vi "SubVI_IntakePID_teleop.vi"(10 "output range":cluster{"output high":dbl, "output low":dbl}={"output high"=100.0, "output low"=-100.0} {"output low" format="%.2f"; "output high" format="%.2f"}, 11 "PID gains":T1={"proportional gain (Kc)"=1.0, "integral time (Ti, min)"=0.01, "derivative time (Td, min)"=0.0} {"derivative time (Td, min)" format="%.3f"; "integral time (Ti, min)" format="%.3f"; "proportional gain (Kc)" format="%.3f"}) -> ()   [LabVIEW 2017]
uses:
  <vilib>/Rock Robotics/Network Tables/NT Read Number.vi
  <vilib>/addons/control/pid/pid.llb/PID (DBL).vi
  <vilib>/addons/control/pid/NI_PID_pid.lvlib
panel:
  out "x-y":dbl
  out "PIDF output":dbl format="%.2f"
  out "Encoder value":dbl
  out "encoder value/PID output":cluster{"output":dbl, "Distance":dbl, dbl}(graph)
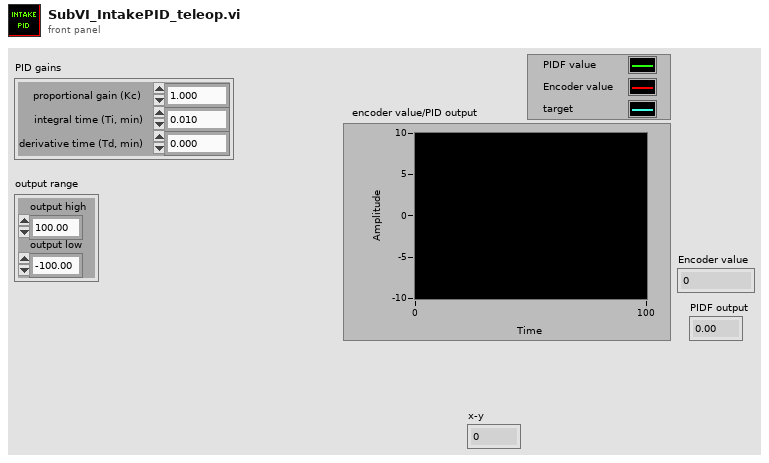
[diagram p1: front panel]
types:
  T1 = cluster{"proportional gain (Kc)":dbl, "integral time (Ti, min)":dbl, "derivative time (Td, min)":dbl}
  T2 = typedef "WPI_EncoderDevRef.ctl" = cluster{"DevStatus":errorcluster, "EncoderIndex":T3, "CounterIndex":T4, "DistancePerCount":dbl, "Decoding Type":T5}
  T3 = typedef "FPGA_EncoderIdx.ctl" = enum8{"Enc 0", "Enc 1", "Enc 2", "Enc 3", "Enc 4", "Enc 5", "Enc 6", "Enc 7", "Invalid"}
  T4 = typedef "FPGA_CounterCtrSystemIndex.ctl" = enum8{"Ctr 0", "Ctr 1", "Ctr 2", "Ctr 3", "Ctr 4", "Ctr 5", "Ctr 6", "Ctr 7", "Invalid"}
  T5 = typedef "WPI_EncoderType.ctl" = enum16{"1x", "2x", "4x"}
  T6 = typedef "WPI_MotorControlDeviceRef.ctl" = cluster{"DeviceStatus":errorcluster, "Type":T7, "PWM":cluster{"PWM Channel":T8, "DeadBand":T9}, "CAN":cluster{"Device Number":u8, "SetOutput VI Ref":variant, "GetOutput VI Ref":variant, "Enable VI Ref":variant, "Disable VI Ref":variant, "Data":variant}, "Invert":bool, "DIO PWM":cluster{"PWM \"Enable\" Channel":T8, "DIOChannel":T10, "PWM Rate":dbl}}
  T7 = typedef "WPI_MotorControlType.ctl" = enum16{"PWM", "CAN", "DIO PWM"}
  T8 = typedef "FPGA_DIOPWMChannel.ctl" = enum8{"PWM 0", "PWM 1", "PWM 2", "PWM 3", "PWM 4", "PWM 5", "PWM 6", "PWM 7", "PWM 8", "PWM 9", "PWM MXP 0", "PWM MXP 1", "PWM MXP 2", "PWM MXP 3", "PWM MXP 4", "PWM MXP 5", "PWM MXP 6", "PWM MXP 7", "PWM MXP 8", "PWM MXP 9", "Invalid"}
  T9 = typedef "WPI_PWMDeadband.ctl" = cluster{"Name":string, "maxPositivePwm":i32, "minPositivePwm":i32, "centerPwm":i32, "maxNegativePwm":i32, "minNegativePwm":i32, "angularRange":u16}
  T10 = typedef "FPGA_DIOChannel.ctl" = enum8{"DIO 0", "DIO 1", "DIO 2", "DIO 3", "DIO 4", "DIO 5", "DIO 6", "DIO 7", "DIO 8", "DIO 9", "DIO MXP 0", "DIO MXP 1", "DIO MXP 2", "DIO MXP 3", "DIO MXP 4", "DIO MXP 5", "DIO MXP 6", "DIO MXP 7", "DIO MXP 8", "DIO MXP 9", "DIO MXP 10", "DIO MXP 11", "DIO MXP 12", "DIO MXP 13", "DIO MXP 14", "DIO MXP 15", "SPI Port CS1", "SPI Port CS2", "SPI Port CS3", "SPI Port MISO", "SPI Port MOSI", "Invalid"}
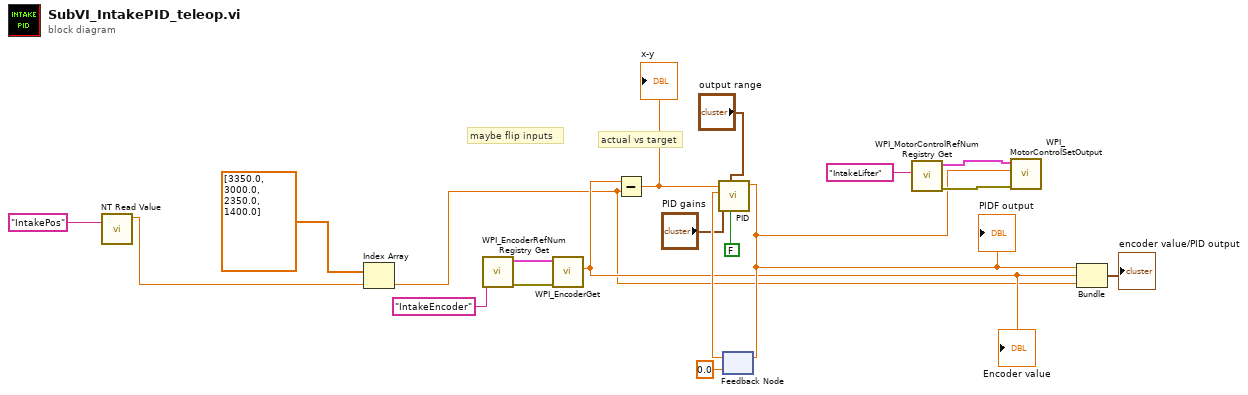
[diagram p0: block diagram]
diagram:
  # "maybe flip inputs"
  # "actual vs target"
  n1 = call-poly <vilib>:"NT Read Value.vi"("Name"="IntakePos") -> ("Numeric"=w6:dbl)  [unwired: 9 in, 1 out]
  n2 = Index Array(array=dbl[] [3350.0, 3000.0, 2350.0, 1400.0], index=w6) -> (element=w1:dbl)
  n3 = call <vilib>:"WPI_EncoderRefNum Registry Get.vi"("refnum name"="IntakeEncoder") -> ("error out"=w9:errorcluster, "EncoderDevRef"=w8:T2)  [unwired: 9 in]
  n4 = call <vilib>:"WPI_EncoderGet.vi"("error in (no error)"=w9, "EncoderDevRef"=w8) -> ("Distance"=w3:dbl)  [unwired: 4 in, 5 out]
  "Encoder value" <- w3
  n5 = Subtract(x=w3, y=w1) -> (x-y=w11:dbl)
  "x-y" <- w11
  n6 = feedback #1(0.0 ("output")) -> (w14:dbl)
  n7 = call-poly <vilib>:"PID.vi"("reinitialize? (F)"=FALSE, "output range"="output range", "PID gains"="PID gains", "process variable"=w14, "setpoint"=w11) -> ("output"=w4:dbl)  [unwired: 5 in, 1 out]
  "PIDF output" <- w4
  n8 = feedback-in #1(w4) -> ()
  n9 = call <vilib>:"WPI_MotorControlRefNum Registry Get.vi"("refnum name"="IntakeLifter") -> ("error out"=w19:errorcluster, "MotorControlDevRef"=w18:T6)  [unwired: 9 in]
  n10 = call <vilib>:"WPI_MotorControlSetOutput.vi"("error in (no error)"=w19, "Output"=w4, "MotorControlDevRef"=w18) -> ()  [unwired: 6 in, 3 out]
  n11 = Bundle("output"=w4, "Distance"=w3, w1) -> (→"encoder value/PID output":cluster{"output":dbl, "Distance":dbl, dbl})  [unwired: 1 in]
